vi "macro_MecaWheelSpeedNormalize.vi"   [LabVIEW 2019, in "Trajectory_Library.lvlib"]
uses:
  Trajectory_Library.lvlib
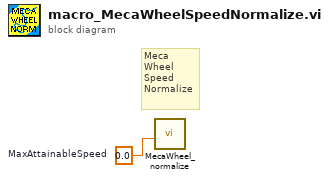
[diagram p0: block diagram]
diagram:
  w1 = 0.0  # MaxAttainableSpeed
  # "Meca\nWheel\nSpeed\nNormalize"
  n1 = call "MecaWheel_normalize.vi"("MaxAttainableSpeed"=w1) -> ()  [unwired: 10 in, 1 out]
